vi "Database Recordset AddNew.vi"(8 "error in (no error)":errorcluster caption="错误输入（无错误）", 9 "Values":variant, 10 "FieldList":variant, 11 "Database Recordset 输入":refnum<class "Database Recordset.lvclass"> caption="DNL_LabVIEW Object in") -> (0 "error out":errorcluster caption="错误输出", 3 "Database Recordset 输出":refnum<class "Database Recordset.lvclass"> caption="DNL_LabVIEW Object out")   [LabVIEW 2011, in "Database Recordset.lvclass"]
uses:
  Database Recordset.lvclass
  Database Recordset.lvclass/Database Recordset.ctl
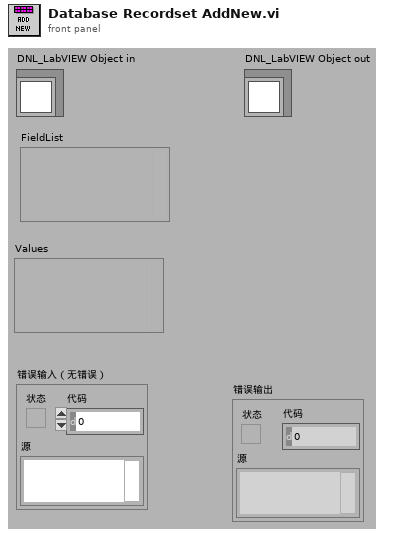
[diagram p1: front panel]
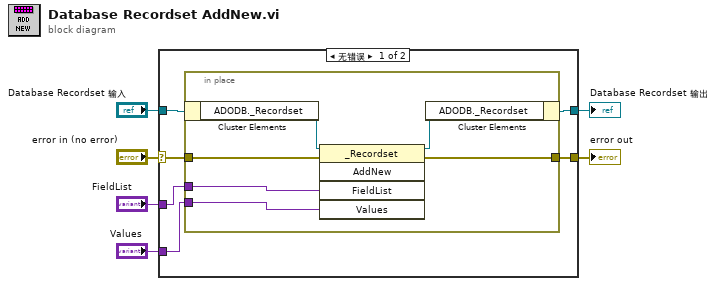
[diagram p0: block diagram]
diagram:
  n1 = case shown="无错误" "error in (no error)" {
    selector: "error in (no error)" -> [w10 w20]
    tunnel: [w9 w20] -> w5
    tunnel: [w11 w19] -> w3
    tunnel: "Database Recordset 输入" -> [w12 w19]
    tunnel: "FieldList" -> [w8 _]
    tunnel: "Values" -> [w7 _]
    frame No Error {
      n2 = in-place {
        in-place-border: w10 -> [w16]
        in-place-border: [w15] -> w9
        in-place-border: w8 -> [w14]
        in-place-border: w7 -> [w13]
        n3 = in-place-cluster #1(w12) -> ("ADODB._Recordset"=w18:refnum<k7>)
        n4 = invoke class="_Recordset" method="AddNew"(reference=w18, error in=w16, "FieldList"=w14, "Values"=w13) -> (reference out=w17:refnum<k7>, error out=w15:errorcluster)  [unwired: 1 in, 3 out]
        n5 = in-place-cluster #1("ADODB._Recordset"=w17) -> (w11:refnum<class "Database Recordset.lvclass">)
      }
    }
    frame Error {
    }
  }
  "error out" <- w5
  "Database Recordset 输出" <- w3
